vi "HEUI_Display_Blink_to_Care.vi"(7 "HEUI_Display_Blink":T2) -> (8 "Care?":T1)   [LabVIEW 2016, in "TLMB.lvlib"]
uses:
  Projects/TLMB.lvlib
  controls/HEUI_Display_Blink.ctl
  controls/HEUI_Display_Care.ctl
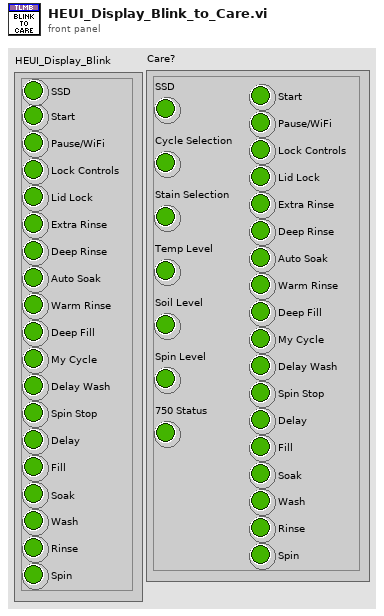
[diagram p1: front panel]
types:
  T1 = typedef "TLMB.lvlib/HEUI_Display_Care.ctl" = cluster{"SSD":bool, "Cycle Selection":bool, "Stain Selection":bool, "Temp Level":bool, "Soil Level":bool, "Spin Level":bool, "750 Status":bool, "Start":bool, "Pause/WiFi":bool, "Lock Controls":bool, "Lid Lock":bool, "Extra Rinse":bool, "Deep Rinse":bool, "Auto Soak":bool, "Warm Rinse":bool, "Deep Fill":bool, "My Cycle":bool, "Delay Wash":bool, "Spin Stop":bool, "Delay":bool, "Fill":bool, "Soak":bool, "Wash":bool, "Rinse":bool, "Spin":bool}
  T2 = typedef "TLMB.lvlib/HEUI_Display_Blink.ctl" = cluster{"Start":bool, "Pause/WiFi":bool, "Lock Controls":bool, "Lid Lock":bool, "Extra Rinse":bool, "Deep Rinse":bool, "Auto Soak":bool, "Warm Rinse":bool, "Deep Fill":bool, "My Cycle":bool, "Delay Wash":bool, "Spin Stop":bool, "Delay":bool, "Fill":bool, "Soak":bool, "Wash":bool, "Rinse":bool, "Spin":bool, "SSD":bool}
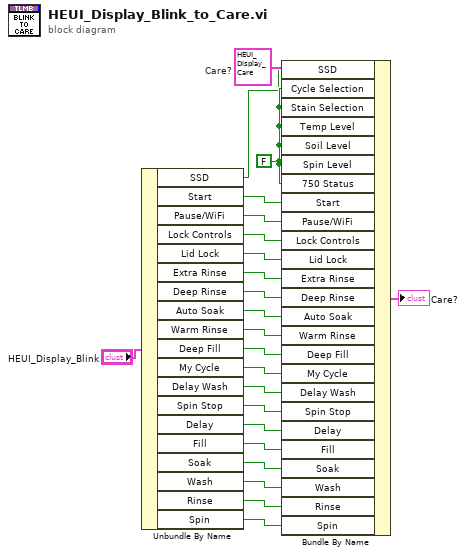
[diagram p0: block diagram]
diagram:
  w9 = T1 {"SSD"=FALSE, "Cycle Selection"=FALSE, "Stain Selection"=FALSE, "Temp Level"=FALSE, "Soil Level"=FALSE, "Spin Level"=FALSE, "750 Status"=FALSE, "Start"=FALSE, "Pause/WiFi"=FALSE, "Lock Controls"=FALSE, "Lid Lock"=FALSE, "Extra Rinse"=FALSE, "Deep Rinse"=FALSE, "Auto Soak"=FALSE, "Warm Rinse"=FALSE, "Deep Fill"=FALSE, "My Cycle"=FALSE, "Delay Wash"=FALSE, "Spin Stop"=FALSE, "Delay"=FALSE, "Fill"=FALSE, "Soak"=FALSE, "Wash"=FALSE, "Rinse"=FALSE, "Spin"=FALSE}  # Care?
  w2 = FALSE
  n1 = Unbundle By Name("HEUI_Display_Blink") -> ("SSD"=w1:bool, "Start"=w22:bool, "Pause/WiFi"=w21:bool, "Lock Controls"=w20:bool, "Lid Lock"=w19:bool, "Extra Rinse"=w18:bool, "Deep Rinse"=w17:bool, "Auto Soak"=w16:bool, "Warm Rinse"=w15:bool, "Deep Fill"=w14:bool, "My Cycle"=w13:bool, "Delay Wash"=w12:bool, "Spin Stop"=w11:bool, "Delay"=w3:bool, "Fill"=w4:bool, "Soak"=w5:bool, "Wash"=w6:bool, "Rinse"=w7:bool, "Spin"=w8:bool)
  n2 = Bundle By Name(cluster=w9, "SSD"=w1, "Cycle Selection"=w2, "Stain Selection"=w2, "Temp Level"=w2, "Soil Level"=w2, "Spin Level"=w2, "750 Status"=w2, "Start"=w22, "Pause/WiFi"=w21, "Lock Controls"=w20, "Lid Lock"=w19, "Extra Rinse"=w18, "Deep Rinse"=w17, "Auto Soak"=w16, "Warm Rinse"=w15, "Deep Fill"=w14, "My Cycle"=w13, "Delay Wash"=w12, "Spin Stop"=w11, "Delay"=w3, "Fill"=w4, "Soak"=w5, "Wash"=w6, "Rinse"=w7, "Spin"=w8) -> (→"Care?":T1)
